vi "3017-1.vi"() -> ()   [LabVIEW 2017]
doc: "I. Description:\nThis example demonstrates how to generate a finite retriggerable digital pulse train from a Counter to be used as the clock for Analog Input. This example utilizes two counters.\n\nII. Instructions for Running:\n1. Select the physical channel to correspond to where your signal is input on the DAQ device.\n2. Enter the minimum and maximum signal ranges.\nNote: For better accuracy, try to match the input range to the expected voltage level of the measured signal.\n3. Select the Counter Channel which corresponds to the counter you want to generate your AI clock from.\n4. Select the Source of the Clock for the acquisition as the output of the counter you chose in step 3.\n5. Set the Rate at which the counter will generate.\nNote: The Rate should be at least twice as fast as the maximum frequency component of the signal being acquired.\n6. Enter the number of Samples per Channel to acquire. This will also be the number of pulses generated by the counter.\n7. Select the Source of the Digital Start Trigger for the acquisition.\n8. Select the edge, rising or falling, on which to trigger.\n\nIII. Block Diagram Steps:\n1. Create an analog input voltage channel. Also, create a Counter Output channel to produce a Pulse in terms of Frequency. If the Idle State of the pulse is set to low the first transition of the generated signal is from low to high.\n2. Define the parameters for an External Clock Source. Additionally, define the sample mode to be continuous. Also, use the DAQmx Timing VI (Implicit) to configure the duration of the pulse generation and the number of pulses to generate.\n3. Use the DAQmx Trigger VI to configure a counter trigger to start on a digital edge.\n4. Configure a buffer which is 1000 plus the number of samples per channel. This is necessary when simulating retriggerable finite transfers with a continuous acquisition because DMA needs a slightly larger buffer than the Samples per Channel. \n5. Use a DAQmx Trigger Property Node to set the operation for retriggerable.\n6. Call the Start VI to begin the acquisition and to arm the counter which begins the pulse train generation.\n7. Use the DAQ Read property node --> AvailSampPerChan to see how many samples have been acquired. If 'Samples per Channel' number of samples have been acquired, as you can set on the front panel, then Read the data, otherwise continue looping. This allows the user to stop the program by pressing the 'STOP' button at any time. \n8. Read the waveform data in a loop until the user hits the stop button or an error occurs.\nNote: This example reads data from one or more channels and returns an array of data. Use the Index Array function to access an individual channel of data.\n9. Call the Clear Task VI to clear the counter Task.\n10. Call the Clear Task VI to clear the AI Task.\n11. Use the popup dialog box to display an error if any.\n\nIV. I/O Connections Overview:\nMake sure your signal input terminal matches the Physical Channel I/O control. Note that there is no external wiring necessary to connect the counter output to the AI clock input. For further connection information, refer to your hardware reference manual."
uses:
  <vilib>/Utility/error.llb/DialogType.ctl
  <vilib>/DAQmx/read.llb/DAQmx Read (Analog 1D Wfm NChan NSamp).vi
  <vilib>/DAQmx/create/channels.llb/DAQmx Create Channel (AI-Voltage-Basic).vi
  <vilib>/DAQmx/configure/timing.llb/DAQmx Timing (Sample Clock).vi
  <vilib>/DAQmx/create/channels.llb/DAQmx Create Channel (CO-Pulse Generation-Frequency).vi
  <vilib>/DAQmx/configure/timing.llb/DAQmx Timing (Implicit).vi
  <vilib>/DAQmx/configure/trigger.llb/DAQmx Start Trigger (Digital Edge).vi
  <vilib>/DAQmx/miscellaneous.llb/DAQmx Fill In Error Info.vi
  <resource>/objmgr/daqmx.rc
panel:
  in  "Stop":bool caption="stop"
  out "Measurement":waveform(dbl)[](graph)
  in  "Clock Source":tag="/Dev1/Ctr0InternalOutput" caption="source"
  in  "Maximum Value":dbl=10.0 format="%0.2f"
  in  "Minimum Value":dbl=-10.0 format="%0.2f"
  in  "Physical Channel":tag="Dev1/ai0"
  in  "Trigger Edge":i32(ring)=10280 items=["Rising"=10280, "Falling"=10171]
  in  "Source":tag="/Dev1/PFI0" caption="Trigger Source"
  in  "Rate (Hz)":dbl=10000.0 format="%0.2f"
  in  "Counter Channel":tag="Dev1/ctr0"
  in  "Samples per Channel":u32=1000
  # "For instructions, select Help>>Show Context Help"
  # "Channel Parameters"
  # "Timing Parameters"
  # "Trigger Parameters"
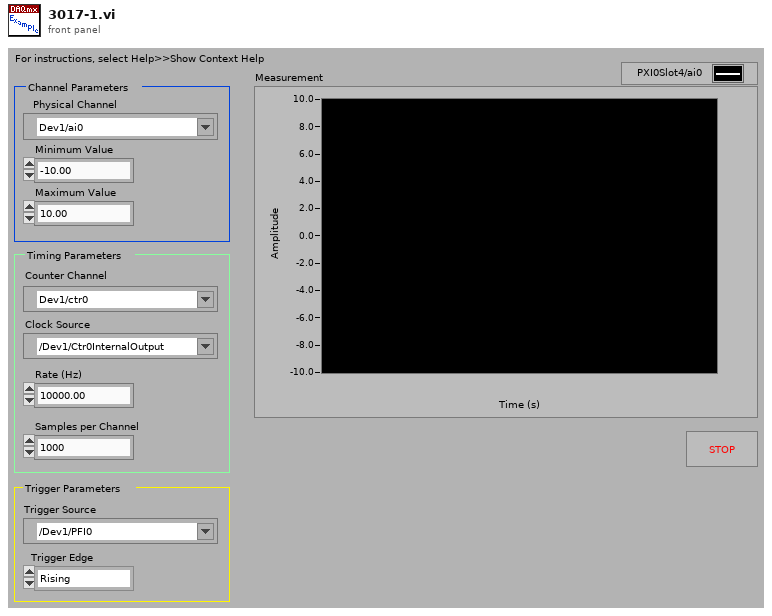
[diagram p1: front panel]
types:
  T1 = typedef "DialogType.ctl" = u16
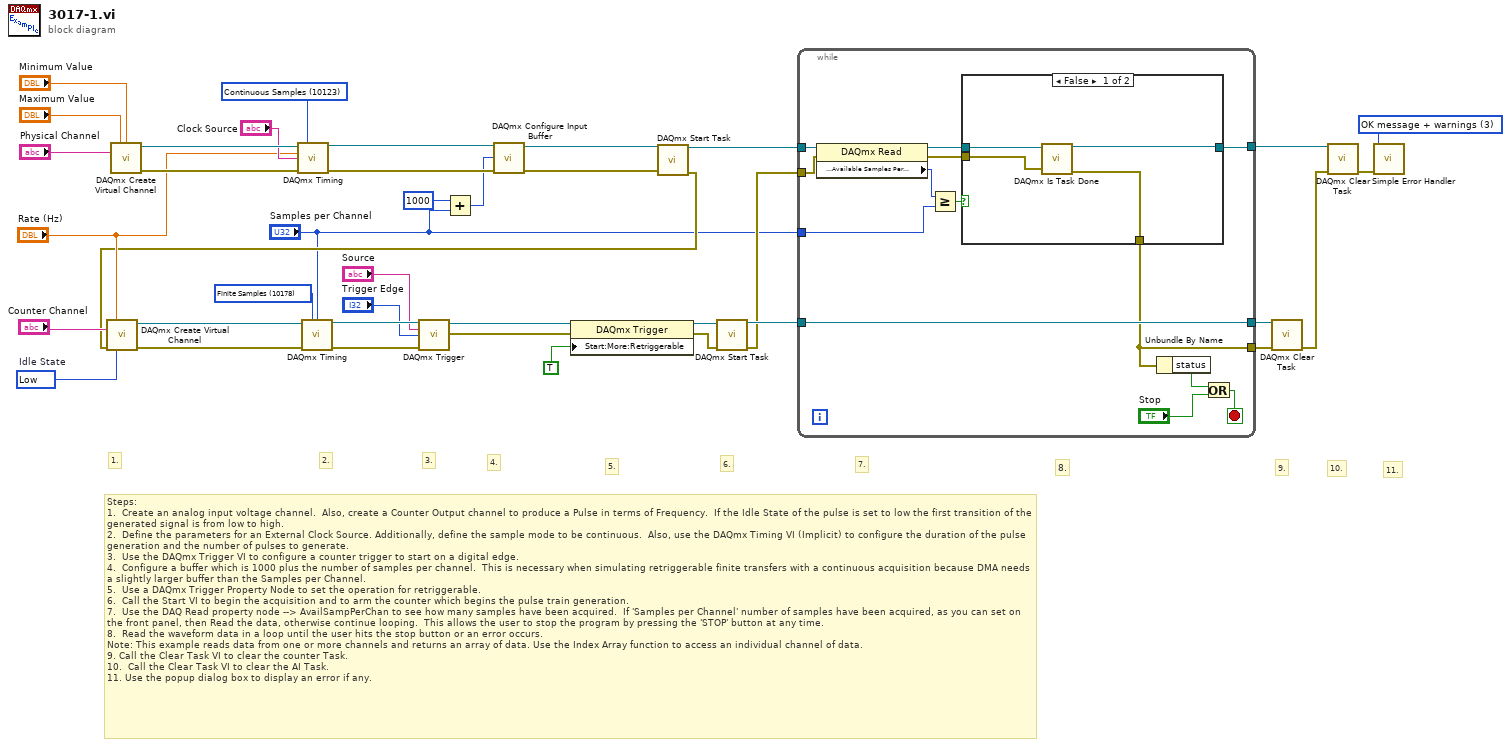
[diagram p0: block diagram]
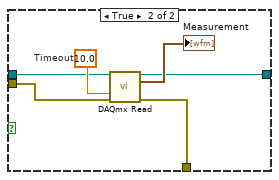
[diagram p2: hidden frame]
diagram:
  w10 = T1 3 items=["no dialog", "OK message", "continue or stop message", "OK message + warnings", "continue/stop + warnings"] ("type of dialog (OK msg:1)")
  w35 = 10214 items=["High"=10192, "Low"=10214]  # Idle State
  w20 = 10123 items=["Finite Samples"=10178, "Continuous Samples"=10123] ("sample mode")
  w37 = 10178 items=["Finite Samples"=10178, "Continuous Samples"=10123] ("sample mode")
  # "11."
  # "6."
  # "7."
  # "10."
  # "2."
  # "1."
  # "9."
  # "5."
  # "8."
  # "4."
  # "Steps: \n1.  Create an analog input voltage channel.  Also, create a Counter Output channel to produce a Pulse in terms of Frequency.  If the Idle State of the pulse is set to low the first transition of the generated signal is from low to high.\n2.  Define the parameters for an External Clock Source. Additionally, define the sample mode to be continuous.  Also, use the DAQmx Timing VI (Implicit) to configure the duration of the pulse generation and the number of pulses to generate.\n3.  Use the DAQmx Trigger VI to configure a counter trigger to start on a digital edge.\n4.  Configure a buffer which is 1000 plus the number of samples per channel.  This is necessary when simulating retriggerable finite transfers with a continuous acquisition because DMA needs a slightly larger buffer than the Samples per Channel. \n5.  Use a DAQmx Trigger Property Node to set the operation for retriggerable.\n6.  Call the Start VI to begin the acquisition and to arm the counter which begins the pulse train generation.\n7.  Use the DAQ Read property node --> AvailSampPerChan to see how many samples have been acquired.  If 'Samples per Channel' number of samples have been acquired, as you can set on the front panel, then Read the data, otherwise continue looping.  This allows the user to stop the program by pressing the 'STOP' button at any time. \n8.  Read the waveform data in a loop until the user hits the stop button or an error occurs.\nNote: This example reads data from one or more channels and returns an array of data. Use the Index Array function to access an individual channel of data.\n9. Call the Clear Task VI to clear the counter Task.\n10.  Call the Clear Task VI to clear the AI Task.\n11. Use the popup dialog box to display an error if any."
  # "3."
  n1 = call-poly <vilib>:"DAQmx Create Virtual Channel.vi"("maximum value"="Maximum Value", "minimum value"="Minimum Value", "physical channels"="Physical Channel") -> ("task out"=w22:refnum<k21>, "error out"=w23:errorcluster)  [unwired: 11 in]
  n2 = call-poly <vilib>:"DAQmx Timing.vi"("task/channels in"=w22, "sample mode"=w20, "rate"="Rate (Hz)", "source"="Clock Source", "error in"=w23) -> ("task out"=w7:refnum<k21>, "error out"=w6:errorcluster)  [unwired: 9 in]
  n3 = Add(x=u32 1000, y="Samples per Channel") -> (x+y=w1:u32)
  n4 = call <vilib>:"DAQmx Configure Input Buffer.vi"("task/channels in"=w7, "buffer size (in samples per channel)"=w1, "error in"=w6) -> ("task out"=w5:refnum<k21>, "error out"=w4:errorcluster)  [unwired: 11 in]
  n5 = call <vilib>:"DAQmx Start Task.vi"("task/channels in"=w5, "error in"=w4) -> ("task out"=w12:refnum<k21>, "error out"=w9:errorcluster)  [unwired: 12 in]
  n6 = call-poly <vilib>:"DAQmx Create Virtual Channel.vi"("frequency"="Rate (Hz)", "counter"="Counter Channel", "error in"=w9, "idle state"=w35) -> ("task out"=w38:refnum<k21>, "error out"=w39:errorcluster)  [unwired: 10 in]
  n7 = call-poly <vilib>:"DAQmx Timing.vi"("task/channels in"=w38, "sample mode"=w37, "samples per channel"="Samples per Channel", "error in"=w39) -> ("task out"=w34:refnum<k21>, "error out"=w33:errorcluster)  [unwired: 10 in]
  n8 = call-poly <vilib>:"DAQmx Trigger.vi"("task/channels in"=w34, "source"="Source", "edge"="Trigger Edge", "error in"=w33) -> ("task out"=w29:refnum<k21>, "error out"=w28:errorcluster)  [unwired: 10 in]
  n9 = property class="DAQmx Trigger"(reference=w29, error in=w28, "Start:More:Retriggerable"=TRUE) -> (reference out=w27:refnum<k21>, error out=w26:errorcluster)
  n10 = call <vilib>:"DAQmx Start Task.vi"("task/channels in"=w27, "error in"=w26) -> ("task out"=w17:refnum<k21>, "error out"=w8:errorcluster)  [unwired: 12 in]
  n11 = while {
    tunnel: w12 -> [w46]
    tunnel: [w48] -> w11
    tunnel: w8 -> [w43]
    tunnel: [w49] -> w16
    tunnel: w17 -> [w49]
    tunnel: [w47] -> w15
    tunnel: "Samples per Channel" -> [w41]
    stop <- w51 stop-if-true
    n12 = property class="DAQmx Read"(reference=w46, error in=w43) -> (reference out=w45:refnum<k21>, error out=w44:errorcluster, "Status:Available Samples Per Channel"=w42:u32)
    n13 = Greater Or Equal?(x=w42, y=w41) -> (x >= y?=w40:bool)
    n14 = case shown="False" w40 {
      tunnel: [w53 w61] -> w48
      tunnel: [w54 w60] -> w47
      tunnel: w45 -> [w56 w58]
      tunnel: w44 -> [w55 w57]
      frame False {
        n15 = call <vilib>:"DAQmx Is Task Done.vi"("task/channels in"=w56, "error in"=w55) -> ("task out"=w53:refnum<k21>, "error out"=w54:errorcluster)  [unwired: 11 in, 1 out]
      }
      frame True {
        w59 = 10.0  # Timeout
        n16 = call-poly <vilib>:"DAQmx Read.vi"("task/channels in"=w58, "timeout"=w59, "error in"=w57) -> ("task out"=w61:refnum<k21>, "data"=→"Measurement":waveform(dbl)[], "error out"=w60:errorcluster)  [unwired: 10 in]
      }
    }
    n17 = Unbundle By Name(w47) -> ("status"=w50:bool)
    n18 = Or(x=w50, y="Stop") -> (x .or. y?=w51:bool)
  }
  n19 = call <vilib>:"DAQmx Clear Task.vi"("task in"=w16, "error in"=w15) -> ("error out"=w14:errorcluster)  [unwired: 13 in]
  n20 = call <vilib>:"DAQmx Clear Task.vi"("task in"=w11, "error in"=w14) -> ("error out"=w13:errorcluster)  [unwired: 13 in]
  n21 = call <vilib>:"Simple Error Handler.vi"("type of dialog (OK msg:1)"=w10, "error in (no error)"=w13) -> ()  [unwired: 3 in, 5 out]
